vi "Load Theme.vi"(8 "Error In":errorcluster, 10 "Theme File Path":path, 11 "ini Theme in":refnum<class "ini Theme.lvclass">) -> (0 "Error Out":errorcluster, 3 "ini Theme out":refnum<class "ini Theme.lvclass">)   [LabVIEW 2021, in "Appearance Actor.lvlib" / "ini Theme.lvclass"]
uses:
  ini Theme.lvclass
  C:/Users/Thomas/Documents/Projects/TemplateVIEW/Sources/Appearance Actor/Theme Classes/Generic Theme/Generic Theme.lvclass
  ini Theme.lvclass/ini Theme.ctl
  Generic Theme/Generic Theme.lvclass/Generic Theme.ctl
  <vilib>/Utility/config.llb/NI_LVConfig.lvlib
  Generic Theme/Generic Theme.lvclass
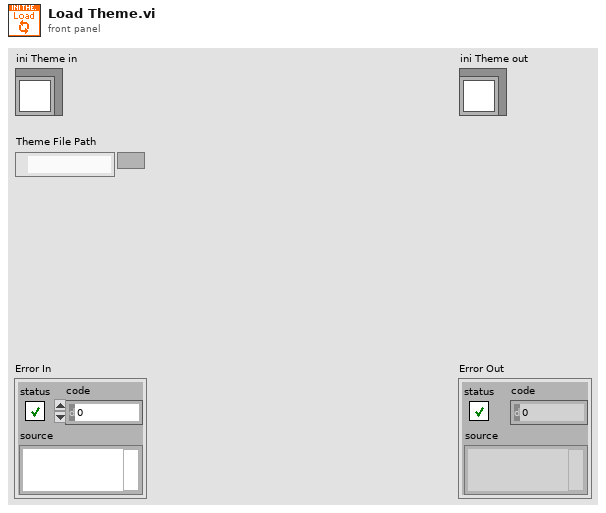
[diagram p1: front panel]
types:
  T1 = typedef "NI_LVConfig.lvlib/Config Data RefNum.ctl" = refnum<k1>
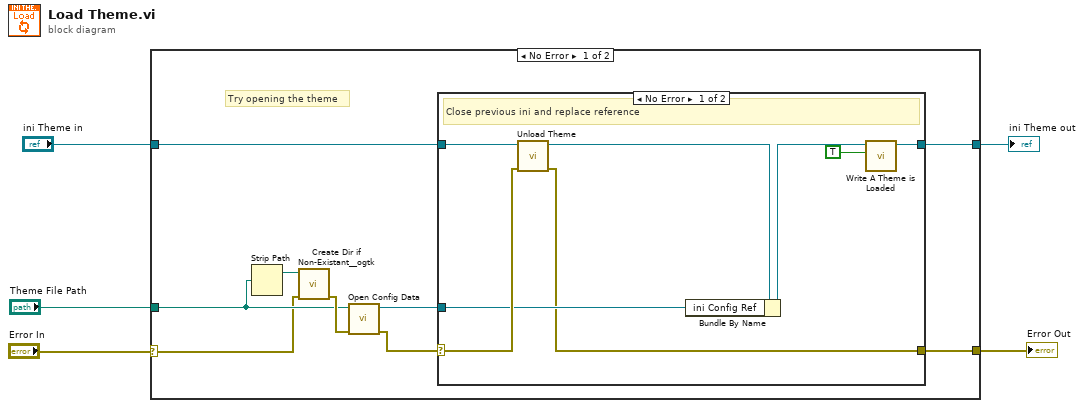
[diagram p0: block diagram]
diagram:
  n1 = case shown="No Error" "Error In" {
    selector: "Error In" -> [w10 w25]
    tunnel: "ini Theme in" -> [w11 w26]
    tunnel: [w8 w25] -> w3
    tunnel: "Theme File Path" -> [w12 _]
    tunnel: [w6 w26] -> w1
    frame No Error {
      # "Try opening the theme"
      n2 = Strip Path(path=w12) -> (stripped path=w13:path)  [unwired: 1 out]
      n3 = call <userlib>:"Create Dir if Non-Existant__ogtk.vi"("error in (no error)"=w10, "Directory Path"=w13) -> ("error out"=w14:errorcluster)  [unwired: 7 in, 2 out]
      n4 = call <vilib>:"Open Config Data.vi"("error in (no error)"=w14, "configuration file path"=w12) -> ("error out"=w9:errorcluster, "refnum"=w7:T1)  [unwired: 7 in, 1 out]
      n5 = case shown="No Error" w9 {
        selector: w9 -> [w20 w24]
        tunnel: [w17 w23] -> w6
        tunnel: w11 -> [w21 w23]
        tunnel: [w16 w24] -> w8
        tunnel: w7 -> [w18 _]
        frame No Error {
          # "Close previous ini and replace reference"
          n6 = call-dynamic "Unload Theme.vi"("Error In"=w20, "ini Theme in"=w21) -> ("Error Out"=w16:errorcluster, "ini Theme out"=w22:refnum<class "ini Theme.lvclass">)  [unwired: 8 in]
          n7 = Bundle By Name(cluster=w22, "ini Config Ref"=w18) -> (w19:refnum<class "ini Theme.lvclass">)
          n8 = call "Write A Theme is Loaded.vi"("A Theme is Loaded"=TRUE, "Generic Theme in"=w19) -> ("Generic Theme out"=w17:refnum<class "ini Theme.lvclass">)  [unwired: 8 in, 1 out]
        }
        frame Error {
          # "Error opening ini file, do nothing, keep previous ini if any"
        }
      }
    }
    frame Error {
    }
  }
  "Error Out" <- w3
  "ini Theme out" <- w1
